vi "SQL-选择清空数据库.vi"(0 "computer1":bool, 1 "computer 2":bool, 2 "ADODB._Connection Out":refnum<k7>, 3 "computer 3":bool, 4 "computer 4":bool, 5 "error in (no error)":errorcluster caption="错误输入（无错误）", 6 "type_c":bool, 7 "computer 5":bool, 8 "computer1_message":bool, 10 "type_b":bool) -> (14 "ADODB._Connection Out 2":refnum<k7>, 19 "error out":errorcluster caption="错误输出")   [LabVIEW 2017]
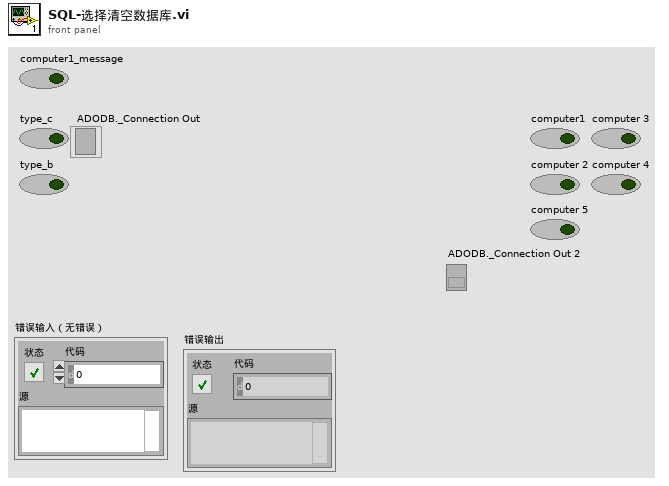
[diagram p1: front panel]
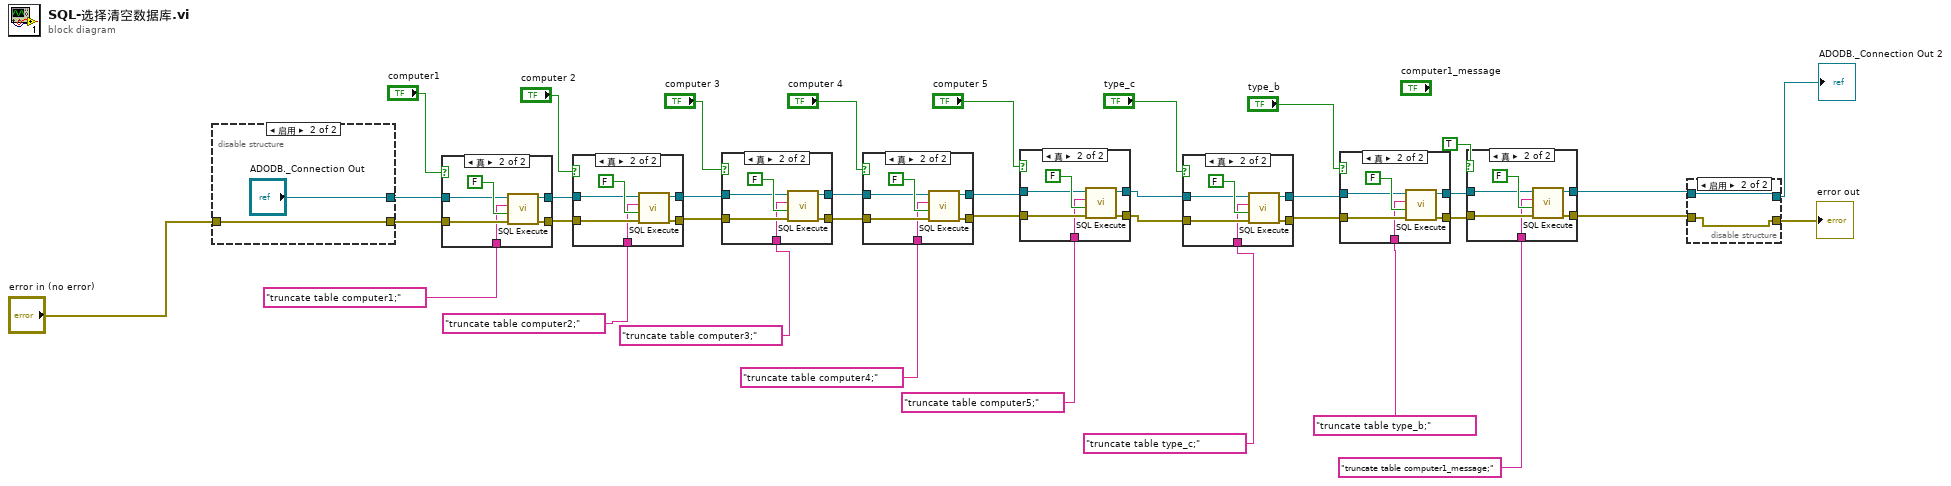
[diagram p0: block diagram]
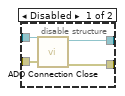
[diagram p3: hidden frame]
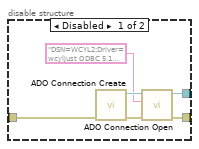
[diagram p4: hidden frame]
diagram:
  n1 = disable-structure shown="启用" {
    disable-tunnel: "error in (no error)" -> [w40 w44]
    disable-tunnel: [w39 "ADODB._Connection Out"] -> w35
    disable-tunnel: [w38 w44] -> w34
    frame Disabled {
      n2 = call <userlib>:"ADO Connection Create.vi"("error in (no error)"=w40) -> ("error out"=w42:errorcluster, "ADODB._Connection Out"=w43:refnum<k7>)  [unwired: 9 in]
      n3 = call <userlib>:"ADO Connection Open.vi"("error in (no error)"=w42, "ConnectionString"="DSN=WCYL2;Driver=wcyljust ODBC 5.1 Driver;UID=root;PWD=root123;", "ADODB._Connection In"=w43) -> ("error out"=w38:errorcluster, "ADODB._Connection Out"=w39:refnum<k7>)  [unwired: 7 in]
    }
    frame Enabled {
    }
  }
  n4 = case shown="真" "computer1" {
    tunnel: [w47 w52] -> w31
    tunnel: [w46 w51] -> w24
    tunnel: w35 -> [w47 w50]
    tunnel: w34 -> [w46 w49]
    tunnel: "truncate table computer1;" ("Command Text") -> [_ w48]
    frame False {
    }
    frame True {
      n5 = call <userlib>:"SQL Execute.vi"("error in (no error)"=w49, "Return Data (T)"=FALSE, "Command Text"=w48, "ADODB._Connection In"=w50) -> ("error out"=w51:errorcluster, "ADODB._Connection Out"=w52:refnum<k7>)  [unwired: 4 in, 2 out]
    }
  }
  n6 = case shown="真" "computer 2" {
    tunnel: [w55 w60] -> w30
    tunnel: [w54 w59] -> w25
    tunnel: w31 -> [w55 w58]
    tunnel: w24 -> [w54 w57]
    tunnel: "truncate table computer2;" ("Command Text") -> [_ w56]
    frame False {
    }
    frame True {
      n7 = call <userlib>:"SQL Execute.vi"("error in (no error)"=w57, "Return Data (T)"=FALSE, "Command Text"=w56, "ADODB._Connection In"=w58) -> ("error out"=w59:errorcluster, "ADODB._Connection Out"=w60:refnum<k7>)  [unwired: 4 in, 2 out]
    }
  }
  n8 = case shown="真" "computer 3" {
    tunnel: [w63 w68] -> w29
    tunnel: [w62 w67] -> w26
    tunnel: w30 -> [w63 w66]
    tunnel: w25 -> [w62 w65]
    tunnel: "truncate table computer3;" ("Command Text") -> [_ w64]
    frame False {
    }
    frame True {
      n9 = call <userlib>:"SQL Execute.vi"("error in (no error)"=w65, "Return Data (T)"=FALSE, "Command Text"=w64, "ADODB._Connection In"=w66) -> ("error out"=w67:errorcluster, "ADODB._Connection Out"=w68:refnum<k7>)  [unwired: 4 in, 2 out]
    }
  }
  n10 = case shown="真" "computer 4" {
    tunnel: [w71 w76] -> w28
    tunnel: [w70 w75] -> w27
    tunnel: w29 -> [w71 w74]
    tunnel: w26 -> [w70 w73]
    tunnel: "truncate table computer4;" ("Command Text") -> [_ w72]
    frame False {
    }
    frame True {
      n11 = call <userlib>:"SQL Execute.vi"("error in (no error)"=w73, "Return Data (T)"=FALSE, "Command Text"=w72, "ADODB._Connection In"=w74) -> ("error out"=w75:errorcluster, "ADODB._Connection Out"=w76:refnum<k7>)  [unwired: 4 in, 2 out]
    }
  }
  n12 = case shown="真" "computer 5" {
    tunnel: [w79 w84] -> w13
    tunnel: [w78 w83] -> w12
    tunnel: w28 -> [w79 w82]
    tunnel: w27 -> [w78 w81]
    tunnel: "truncate table computer5;" ("Command Text") -> [_ w80]
    frame False {
    }
    frame True {
      n13 = call <userlib>:"SQL Execute.vi"("error in (no error)"=w81, "Return Data (T)"=FALSE, "Command Text"=w80, "ADODB._Connection In"=w82) -> ("error out"=w83:errorcluster, "ADODB._Connection Out"=w84:refnum<k7>)  [unwired: 4 in, 2 out]
    }
  }
  n14 = case shown="真" "type_c" {
    tunnel: [w87 w92] -> w14
    tunnel: [w86 w91] -> w15
    tunnel: w13 -> [w87 w90]
    tunnel: w12 -> [w86 w89]
    tunnel: "truncate table type_c;" ("Command Text") -> [_ w88]
    frame False {
    }
    frame True {
      n15 = call <userlib>:"SQL Execute.vi"("error in (no error)"=w89, "Return Data (T)"=FALSE, "Command Text"=w88, "ADODB._Connection In"=w90) -> ("error out"=w91:errorcluster, "ADODB._Connection Out"=w92:refnum<k7>)  [unwired: 4 in, 2 out]
    }
  }
  n16 = case shown="真" "type_b" {
    tunnel: [w95 w100] -> w3
    tunnel: [w94 w99] -> w6
    tunnel: w14 -> [w95 w98]
    tunnel: w15 -> [w94 w97]
    tunnel: "truncate table type_b;" ("Command Text") -> [_ w96]
    frame False {
    }
    frame True {
      n17 = call <userlib>:"SQL Execute.vi"("error in (no error)"=w97, "Return Data (T)"=FALSE, "Command Text"=w96, "ADODB._Connection In"=w98) -> ("error out"=w99:errorcluster, "ADODB._Connection Out"=w100:refnum<k7>)  [unwired: 4 in, 2 out]
    }
  }
  n18 = case shown="真" TRUE {
    tunnel: [w103 w108] -> w4
    tunnel: [w102 w107] -> w5
    tunnel: w3 -> [w103 w106]
    tunnel: w6 -> [w102 w105]
    tunnel: "truncate table computer1_message;" ("Command Text") -> [_ w104]
    frame False {
    }
    frame True {
      n19 = call <userlib>:"SQL Execute.vi"("error in (no error)"=w105, "Return Data (T)"=FALSE, "Command Text"=w104, "ADODB._Connection In"=w106) -> ("error out"=w107:errorcluster, "ADODB._Connection Out"=w108:refnum<k7>)  [unwired: 4 in, 2 out]
    }
  }
  n20 = disable-structure shown="启用" {
    disable-tunnel: [w113 w115] -> w37
    disable-tunnel: w4 -> [w112 w114]
    disable-tunnel: w5 -> [w111 w115]
    disable-tunnel: [w110 w114] -> w7
    frame Disabled {
      n21 = call <userlib>:"ADO Connection Close.vi"("error in (no error)"=w111, "ADODB._Connection In"=w112) -> ("error out"=w113:errorcluster, "ADODB._Connection Out"=w110:refnum<k7>)  [unwired: 8 in]
    }
    frame Enabled {
    }
  }
  "error out" <- w37
  "ADODB._Connection Out 2" <- w7
